vi "FindLVLibProjectPath.vi"(8 "error in (no error)":errorcluster, 10 "SourceFolderPath":path, 11 "SourceFolderPaths":path[](array[path])) -> (0 "error out":errorcluster, 3 "LV Project Not Found []":path[](array[path]))   [LabVIEW 2019]
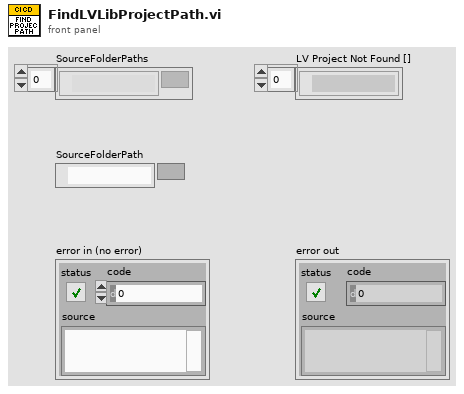
[diagram p1: front panel]
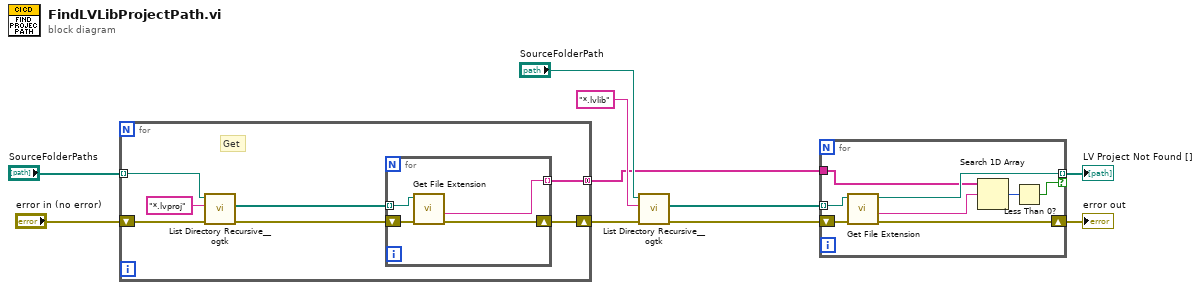
[diagram p0: block diagram]
diagram:
  n1 = for {
    shift-right: [w13] -> w3
    shift-left: "error in (no error)" -> [w17]
    tunnel: "SourceFolderPaths" -> [w12] mode=indexing
    tunnel: [w11] -> w5 mode=concatenating
    # "Get"
    n2 = call <userlib>:"List Directory Recursive__ogtk.vi"("error in (no error)"=w17, "pattern"="*.lvproj", "Path"=w12) -> ("error out"=w16:errorcluster, "file paths"=w15:path[])  [unwired: 5 in, 2 out]
    n3 = for {
      tunnel: w15 -> [w20] mode=indexing
      shift-right: [w19] -> w13
      shift-left: w16 -> [w21]
      tunnel: [w18] -> w11 mode=indexing
      n4 = call <vilib>:"Get File Extension.vi"("error in (no error)"=w21, "file"=w20) -> ("error out"=w19:errorcluster, "filename without extension"=w18:string)  [unwired: 5 in, 3 out]
    }
  }
  n5 = call <userlib>:"List Directory Recursive__ogtk.vi"("error in (no error)"=w3, "pattern"="*.lvlib", "Path"="SourceFolderPath") -> ("error out"=w2:errorcluster, "file paths"=w6:path[])  [unwired: 5 in, 2 out]
  n6 = for {
    tunnel: w6 -> [w28] mode=indexing
    shift-right: [w27] -> w1
    shift-left: w2 -> [w29]
    tunnel: [w26] -> w4 mode=indexing if=w22
    tunnel: w5 -> [w25]
    n7 = call <vilib>:"Get File Extension.vi"("error in (no error)"=w29, "file"=w28) -> ("error out"=w27:errorcluster, "filename without extension"=w24:string, "dup file"=w26:path)  [unwired: 5 in, 2 out]
    n8 = Search 1D Array(1D array=w25, element=w24) -> (index of element=w23:i32)  [unwired: 1 in]
    n9 = Less Than 0?(x=w23) -> (x < 0?=w22:bool)
  }
  "error out" <- w1
  "LV Project Not Found []" <- w4
